vi "6. Informative Queue Based State Machine Traffic Light Simulator.vi"() -> ()   [LabVIEW 2018]
uses:
  Typedefs/Traffic Light States for Queue based example.ctl
panel:
  out "Element\nLast Dequeued":cluster{"Next State":T1, "Wait Time":u32}
  out "Queue":cluster{"Next State":T1, "Wait Time":u32}[](array[cluster])
  in  "stop":bool
  out "Yellow":bool
  out "Green":bool
  out "Red":bool
  out "Traffic Lights Picture":picture
  # "Traffic Light Graphic Vector by Vecteezy\n(https://www.vecteezy.com/free-vector/graphic)"
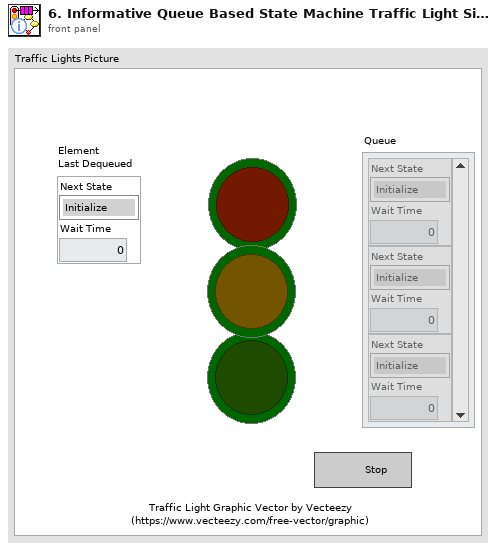
[diagram p1: front panel]
types:
  T1 = typedef "Traffic Light States for Queue based example.ctl" = enum16{"Initialize", "Red", "Yellow", "Green", "Wait", "Stop"}
  T2 = cluster{"Wait Before Red":u32, "Wait Before Yellow":u32, "Wait Before Green":u32}
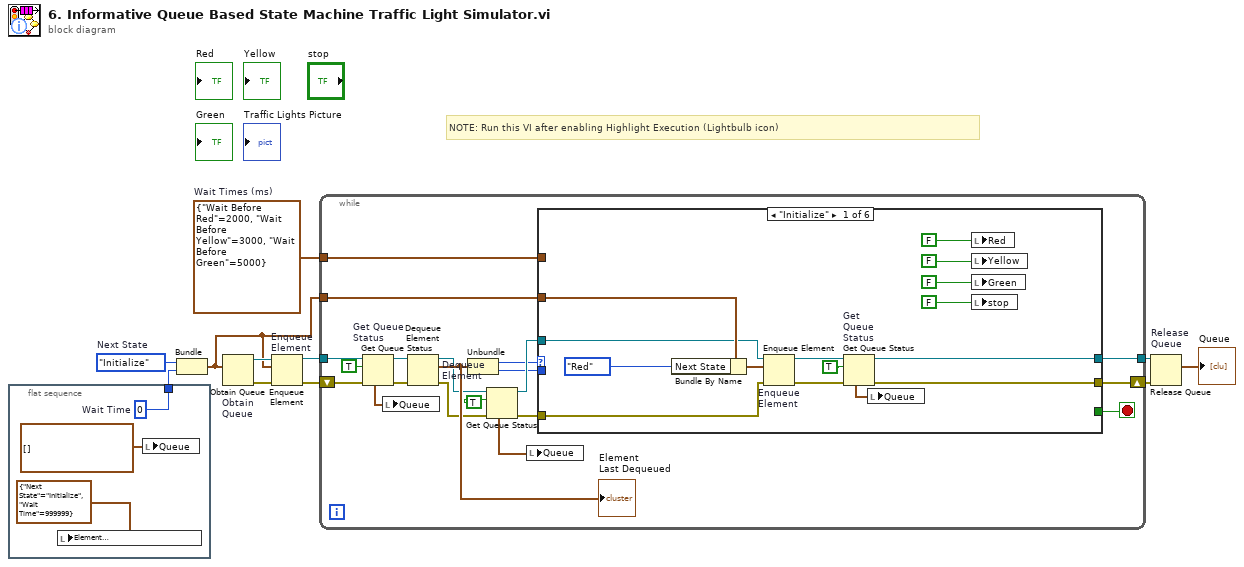
[diagram p0: block diagram]
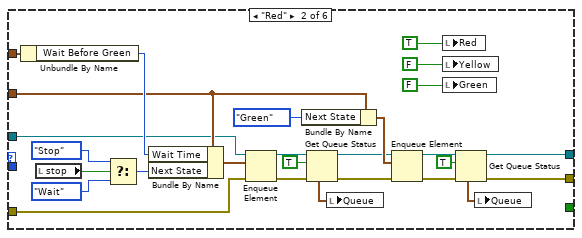
[diagram p2: hidden frame]
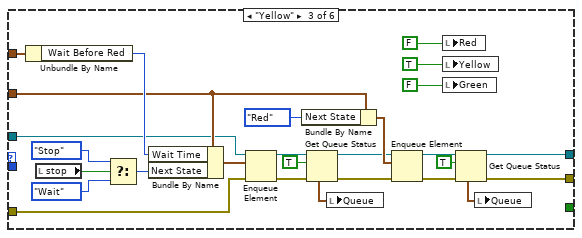
[diagram p3: hidden frame]
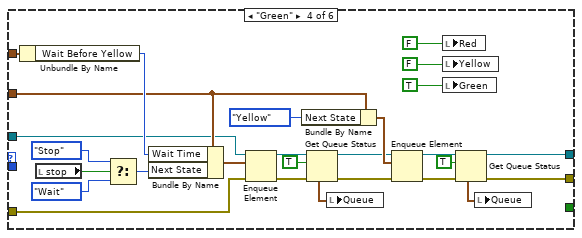
[diagram p4: hidden frame]
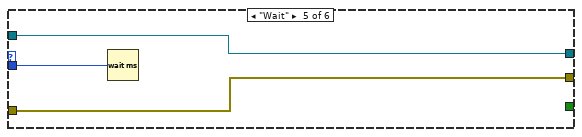
[diagram p5: hidden frame]
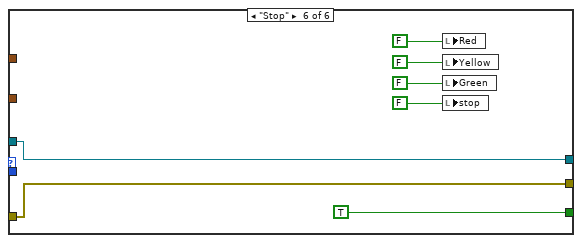
[diagram p6: hidden frame]
diagram:
  w11 = T2 {"Wait Before Red"=2000, "Wait Before Yellow"=3000, "Wait Before Green"=5000}  # Wait Times (ms)
  w10 = Traffic_Light_States_for_Queue_based_example."Initialize"  # Next State
  # "NOTE: Run this VI after enabling Highlight Execution (Lightbulb icon)"
  n1 = flat-sequence {
    tunnel: [w14] -> w9
    frame #0 {
      w14 = u32 0  # Wait Time
      n2 = local write "Element\nLast Dequeued"(cluster{"Next State":T1, "Wait Time":u32} {"Next State"=enum."Initialize", "Wait Time"=999999} ("Element\nLast Dequeued")) -> ()
      n3 = local write "Queue"(cluster{"Next State":T1, "Wait Time":u32}[] [] ("Queue")) -> ()
    }
  }
  n4 = Bundle("Next State"=w10, "Wait Time"=w9) -> (w5:cluster{"Next State":T1, "Wait Time":u32})  [unwired: 1 in]
  n5 = Obtain Queue "Obtain\nQueue"(element data type=w5) -> (queue out=w8:refnum<queue>, error out=w6:errorcluster)  [unwired: 4 in, 1 out]
  n6 = Enqueue Element "Enqueue\nElement"(queue=w8, element=w5, error in (no error)=w6) -> (queue out=w7:refnum<queue>, error out=w4:errorcluster)  [unwired: 1 in, 1 out]
  n7 = while {
    tunnel: w11 -> [w32]
    tunnel: w5 -> [w29]
    shift-right: [w24] -> w3
    shift-left: w4 -> [w26]
    tunnel: w7 -> [w22]
    tunnel: [w28] -> w2
    stop <- w31 stop-if-true
    n8 = Get Queue Status "Get Queue\nStatus"(queue=w22, return elements? (F)=TRUE, error in (no error)=w26) -> (queue out=w21:refnum<queue>, error out=w23:errorcluster, elements=w19:cluster{"Next State":T1, "Wait Time":u32}[])  [unwired: 5 out]
    n9 = local write "Queue"(w19) -> ()
    n10 = Dequeue Element "Dequeue\nElement"(queue=w21, error in (no error)=w23) -> (queue out=w17:refnum<queue>, element=w34:cluster{"Next State":T1, "Wait Time":u32}, error out=w25:errorcluster)  [unwired: 1 in, 1 out]
    "Element\nLast Dequeued" <- w34
    n11 = Unbundle(w34) -> ("Next State"=w30:T1, "Wait Time"=w27:u32)
    n12 = Get Queue Status(queue=w17, return elements? (F)=TRUE, error in (no error)=w25) -> (queue out=w33:refnum<queue>, error out=w18:errorcluster, elements=w15:cluster{"Next State":T1, "Wait Time":u32}[])  [unwired: 5 out]
    n13 = local write "Queue"(w15) -> ()
    n14 = case shown="\"Initialize\"" w30 {
      tunnel: [w35 w52 w79 w106 w133 w140] -> w28
      tunnel: w32 -> [_ w67 w94 w121 _ _]
      tunnel: [_ _ _ _ _ TRUE] -> w31
      tunnel: w29 -> [w45 w65 w92 w119 _ _]
      tunnel: w33 -> [w42 w62 w89 w116 w133 w140]
      tunnel: w27 -> [_ _ _ _ w132 _]
      tunnel: w18 -> [w41 w61 w88 w115 w131 w138]
      tunnel: [w38 w54 w81 w108 w131 w138] -> w24
      frame "Initialize" {
        n15 = Bundle By Name(cluster=w45, "Next State"=Traffic_Light_States_for_Queue_based_example."Red") -> (w43:cluster{"Next State":T1, "Wait Time":u32})
        n16 = Enqueue Element "Enqueue\nElement"(queue=w42, element=w43, error in (no error)=w41) -> (queue out=w36:refnum<queue>, error out=w37:errorcluster)  [unwired: 1 in, 1 out]
        n17 = Get Queue Status "Get\nQueue\nStatus"(queue=w36, return elements? (F)=TRUE, error in (no error)=w37) -> (queue out=w35:refnum<queue>, error out=w38:errorcluster, elements=w40:cluster{"Next State":T1, "Wait Time":u32}[])  [unwired: 5 out]
        n18 = local write "Queue"(w40) -> ()
        n19 = local write "Red"(FALSE ("Red")) -> ()
        n20 = local write "Yellow"(FALSE ("Red")) -> ()
        n21 = local write "Green"(FALSE ("Red")) -> ()
        n22 = local write "stop"(FALSE ("stop")) -> ()
      }
      frame "Red" {
        n23 = Unbundle By Name(w67) -> ("Wait Before Green"=w66:u32)
        n24 = local read "stop"() -> (w69:bool)
        n25 = Select(t=Traffic_Light_States_for_Queue_based_example."Stop" ("Next State"), s=w69, f=Traffic_Light_States_for_Queue_based_example."Wait" ("Next State")) -> (s? t:f=w70:T1)
        n26 = Bundle By Name(cluster=w65, "Wait Time"=w66, "Next State"=w70) -> (w72:cluster{"Next State":T1, "Wait Time":u32})
        n27 = Enqueue Element(queue=w62, element=w72, error in (no error)=w61) -> (queue out=w58:refnum<queue>, error out=w76:errorcluster)  [unwired: 1 in, 1 out]
        n28 = Bundle By Name(cluster=w65, "Next State"=Traffic_Light_States_for_Queue_based_example."Green") -> (w63:cluster{"Next State":T1, "Wait Time":u32})
        n29 = Get Queue Status(queue=w58, return elements? (F)=TRUE, error in (no error)=w76) -> (queue out=w57:refnum<queue>, error out=w59:errorcluster, elements=w55:cluster{"Next State":T1, "Wait Time":u32}[])  [unwired: 5 out]
        n30 = local write "Queue"(w55) -> ()
        n31 = Enqueue Element(queue=w57, element=w63, error in (no error)=w59) -> (queue out=w53:refnum<queue>, error out=w60:errorcluster)  [unwired: 1 in, 1 out]
        n32 = local write "Red"(TRUE ("Red")) -> ()
        n33 = local write "Yellow"(FALSE ("Red")) -> ()
        n34 = local write "Green"(FALSE ("Red")) -> ()
        n35 = Get Queue Status(queue=w53, return elements? (F)=TRUE, error in (no error)=w60) -> (queue out=w52:refnum<queue>, error out=w54:errorcluster, elements=w50:cluster{"Next State":T1, "Wait Time":u32}[])  [unwired: 5 out]
        n36 = local write "Queue"(w50) -> ()
      }
      frame "Yellow" {
        n37 = Unbundle By Name(w94) -> ("Wait Before Red"=w93:u32)
        n38 = local read "stop"() -> (w96:bool)
        n39 = Select(t=Traffic_Light_States_for_Queue_based_example."Stop" ("Next State"), s=w96, f=Traffic_Light_States_for_Queue_based_example."Wait" ("Next State")) -> (s? t:f=w97:T1)
        n40 = Bundle By Name(cluster=w92, "Wait Time"=w93, "Next State"=w97) -> (w99:cluster{"Next State":T1, "Wait Time":u32})
        n41 = Enqueue Element(queue=w89, element=w99, error in (no error)=w88) -> (queue out=w85:refnum<queue>, error out=w103:errorcluster)  [unwired: 1 in, 1 out]
        n42 = Bundle By Name(cluster=w92, "Next State"=Traffic_Light_States_for_Queue_based_example."Red") -> (w90:cluster{"Next State":T1, "Wait Time":u32})
        n43 = Get Queue Status(queue=w85, return elements? (F)=TRUE, error in (no error)=w103) -> (queue out=w84:refnum<queue>, error out=w86:errorcluster, elements=w82:cluster{"Next State":T1, "Wait Time":u32}[])  [unwired: 5 out]
        n44 = local write "Queue"(w82) -> ()
        n45 = Enqueue Element(queue=w84, element=w90, error in (no error)=w86) -> (queue out=w80:refnum<queue>, error out=w87:errorcluster)  [unwired: 1 in, 1 out]
        n46 = local write "Red"(FALSE ("Red")) -> ()
        n47 = local write "Yellow"(TRUE ("Red")) -> ()
        n48 = local write "Green"(FALSE ("Red")) -> ()
        n49 = Get Queue Status(queue=w80, return elements? (F)=TRUE, error in (no error)=w87) -> (queue out=w79:refnum<queue>, error out=w81:errorcluster, elements=w77:cluster{"Next State":T1, "Wait Time":u32}[])  [unwired: 5 out]
        n50 = local write "Queue"(w77) -> ()
      }
      frame "Green" {
        n51 = Unbundle By Name(w121) -> ("Wait Before Yellow"=w120:u32)
        n52 = local read "stop"() -> (w123:bool)
        n53 = Select(t=Traffic_Light_States_for_Queue_based_example."Stop" ("Next State"), s=w123, f=Traffic_Light_States_for_Queue_based_example."Wait" ("Next State")) -> (s? t:f=w124:T1)
        n54 = Bundle By Name(cluster=w119, "Wait Time"=w120, "Next State"=w124) -> (w126:cluster{"Next State":T1, "Wait Time":u32})
        n55 = Enqueue Element(queue=w116, element=w126, error in (no error)=w115) -> (queue out=w112:refnum<queue>, error out=w130:errorcluster)  [unwired: 1 in, 1 out]
        n56 = Bundle By Name(cluster=w119, "Next State"=Traffic_Light_States_for_Queue_based_example."Yellow") -> (w117:cluster{"Next State":T1, "Wait Time":u32})
        n57 = Get Queue Status(queue=w112, return elements? (F)=TRUE, error in (no error)=w130) -> (queue out=w111:refnum<queue>, error out=w113:errorcluster, elements=w109:cluster{"Next State":T1, "Wait Time":u32}[])  [unwired: 5 out]
        n58 = local write "Queue"(w109) -> ()
        n59 = Enqueue Element(queue=w111, element=w117, error in (no error)=w113) -> (queue out=w107:refnum<queue>, error out=w114:errorcluster)  [unwired: 1 in, 1 out]
        n60 = local write "Red"(FALSE ("Red")) -> ()
        n61 = local write "Yellow"(FALSE ("Red")) -> ()
        n62 = local write "Green"(TRUE ("Red")) -> ()
        n63 = Get Queue Status(queue=w107, return elements? (F)=TRUE, error in (no error)=w114) -> (queue out=w106:refnum<queue>, error out=w108:errorcluster, elements=w104:cluster{"Next State":T1, "Wait Time":u32}[])  [unwired: 5 out]
        n64 = local write "Queue"(w104) -> ()
      }
      frame "Wait" {
        n65 = Wait (ms)(milliseconds to wait=w132) -> ()  [unwired: 1 out]
      }
      frame "Stop" {
        n66 = local write "Red"(FALSE ("Red")) -> ()
        n67 = local write "Yellow"(FALSE ("Red")) -> ()
        n68 = local write "Green"(FALSE ("Red")) -> ()
        n69 = local write "stop"(FALSE ("stop")) -> ()
      }
    }
  }
  n70 = Release Queue "Release\nQueue"(queue=w2, error in (no error)=w3) -> (remaining elements=→"Queue":cluster{"Next State":T1, "Wait Time":u32}[])  [unwired: 1 in, 2 out]
